vi "Event Handle Loop_Image Bounds.vi"(1 "Image":T1) -> (0 "Bounds":cluster{"Width":i16, "Height":i16})   [LabVIEW 2020, in "QTab.lvlib" / "QMenu Class.lvclass"]
uses:
  QMenu Class.lvclass
  <vilib>/picture/picture.llb/imagedata.ctl
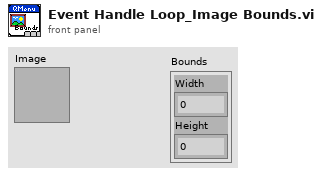
[diagram p1: front panel]
types:
  T1 = typedef "imagedata.ctl" = cluster{"image type":i32, "image depth":i32, "image":u8[], "mask":u8[], "colors":u32[], "Rectangle":cluster{"left":i16, "top":i16, "right":i16, "bottom":i16}}
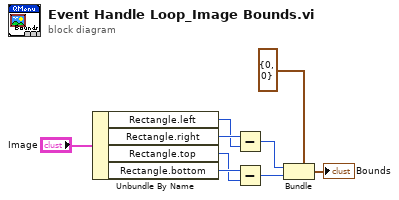
[diagram p0: block diagram]
diagram:
  n1 = Unbundle By Name("Image") -> ("Rectangle.left"=w7:i16, "Rectangle.right"=w8:i16, "Rectangle.top"=w5:i16, "Rectangle.bottom"=w6:i16)
  n2 = Subtract(x=w8, y=w7) -> (x-y=w3:i16)
  n3 = Subtract(x=w6, y=w5) -> (x-y=w4:i16)
  n4 = Bundle(cluster=cluster{"Width":i16, "Height":i16} {"Width"=0, "Height"=0} ("Bounds"), "Width"=w3, "Height"=w4) -> (→"Bounds":cluster{"Width":i16, "Height":i16})
